vi "PAN_SendObsFinish.vi"(7 "command":string="EXPOSE", 8 "error in":errorcluster, 10 "obsID":string, 11 "done queue":refnum<queue>) -> ()   [LabVIEW 2016]
uses:
  private/vis/PAN_ObsFinishStruct.ctl
panel:
  in  "Cluster":T1
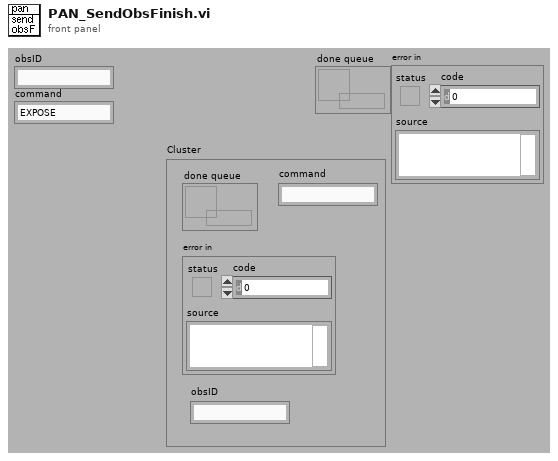
[diagram p1: front panel]
types:
  T1 = typedef "PAN_ObsFinishStruct.ctl" = cluster{"done queue":refnum<queue>, "error in":errorcluster, "obsID":string, "command":string}
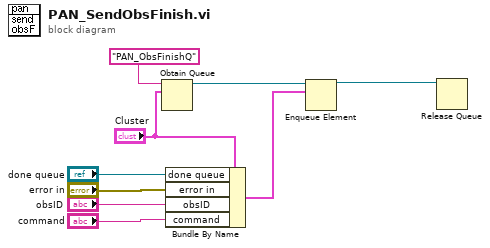
[diagram p0: block diagram]
diagram:
  n1 = Obtain Queue(name (unnamed)="PAN_ObsFinishQ", element data type="Cluster") -> (queue out=w8:refnum<queue>)  [unwired: 3 in, 2 out]
  n2 = Bundle By Name(cluster="Cluster", "done queue"="done queue", "error in"="error in", "obsID"="obsID", "command"="command") -> (w5:T1)
  n3 = Enqueue Element(queue=w8, element=w5) -> (queue out=w7:refnum<queue>)  [unwired: 1 in, 3 out]
  n4 = Release Queue(queue=w7) -> ()  [unwired: 1 in, 4 out]
